vi "RedMoRaceTiming.vi"() -> ()   [LabVIEW 2022 SP3]
uses:
  <vilib>/event_ctls.llb/eventvkey.ctl
  subVIs/BackupFileMgmtStates.ctl
  subVIs/ConfigFileLoopStates.ctl
  <vilib>/Utility/miscctls.llb/LVRowAndColumnUnsignedTypeDef.ctl
  <vilib>/Utility/config.llb/Read Key (I32).vi
  <vilib>/Utility/config.llb/Read Key (Double).vi
  <vilib>/Utility/config.llb/Read Key (Path).vi
  <vilib>/Utility/config.llb/Write Key (Double).vi
  <vilib>/Utility/config.llb/Write Key (I32).vi
  <vilib>/Utility/config.llb/Write Key (Path).vi
  <vilib>/Utility/file.llb/Write Delimited Spreadsheet (string).vi
  <vilib>/Utility/config.llb/NI_LVConfig.lvlib
panel:
  out "Config File Error?":bool
  out "Mode":bool
  out "Event Handler Error?":bool
  out "Backup File Error?":bool
  out "File Mgmt Error?":bool
  out "Finish Table":string[][](table)
  out "Duplicate Bib #s":string[](array[string])
  out "Backup File Saving?":bool
  out "Overall Error Status":bool
  in  "Clear Next Bib":bool
  in  "Bib":string
  out "Race Time":string
  in  "Tab Control":T1(tab)
  out "Racers Remaining":i32
  in  "Enable Button Timing Controls":bool
  out "Duplicate Bib #s":i32
  in  "Bib-Only Button":bool
  in  "Time Only Button":bool
  in  "Control Time Button":bool
  out "Total Times":i32
  out "Total Bibs":i32
  out "Total Control Times":i32
  out "File I/O Error":errorcluster
  out "Backup File I/O Error":errorcluster
  out "Total Racers":i32
  in  "stop":bool
  in  "Time Correction in seconds (increments by .1s)":dbl step=0.1
  out "Overall error out":errorcluster
  in  "Total Racers Control":i32
  in  "Setup/Race Mode Toggle":bool=TRUE
  out "Setup Mode":bool
  out "Race Mode":bool=TRUE
  in  "Save Config File":bool
  in  "CLEAR ARRAYS":bool
  in  "External/Backup Data Path":path=path "D:/RedMoRace"
  in  "SAVE TO FILE":bool
  out "File Path of Main Race File":path
  in  "Enable?":bool=TRUE
  out "Backup File I/O State":T2
  out "ArrayOfControlTimeMarkers":string[](array[string])
  out "VKey":T3
  out "ArrayOfBibs":string[](array[string])
  out "*(type *) &x":string
  out "Char":i16
  out "ArrayOfTimes":string[](array[string])
  # "Red Mo Race Timing\nv2025\nDeveloped by Aaron Fleishman"
  # "Index"
  # "Bib"
  # "Time"
  # "Control Time?"
  # "Statistics"
  # "This is race timing software for downriver canoe and kayak racing. This was designed to operate using a number pad (built-in or USB attachable).\n\nThe software app is able to log three different kinds of data:\n - Time Only - SPACE BAR.\n - Control Time (Bib + Time) - R key\n - Bib only (starting from last control time or last bib, use carefully) - ENTER (on number pad only)"
  # "Timing Controls"
  # "Race Time Correction"
  # "Number of Total Racers Setup"
  # "Errors"
  # "Primary File Management"
  # "External/Backup File Management"
  # "This application is used to assist in timing for the Red Moshannon Downriver Race.\n\n1. Open timing software several minutes prior to finishers and use \"Time/Racer Setup & Errors\" to sync \"Race Time\" in app with official race time stopwatch. Once finishers have crossed the line, do not make any adjustments to time.\n\n2. Configure backup file. The app will store two copies of the race data, one locally and one in a backup location. Typically, the backup location is a remote drive or SD card. This provides backup in case the PC has sudden failure.\n\n3. If known, update the total number of boats racing. This will give you a countdown of total bibs remaining on the main screen.\n\n4. For operations, you need to have multiple spotters. The spotters should have notepads ready to record bib numbers in order that they cross the finish line.\n\n5. As timer, your primary responsbility is to log TIMES. The spotters primary responsbility is to log BIBS in the correct order. After the race, you can merge the two.\n\n6. In order to reduce a single missed value messing all of the data, the timers and spotters should employ \"Control Times\" as frequently as able. Control Times are known correct bib + correct time. If a single boat is crossing with plenty of time before and after, queue the bib number in the box using the number keys, and use the \"R\" key when the boater crosses the line to log a control time. Spotters should also record the time with bib number.\n\n7. After the race, you need to go back and fill in the gaps between Control Times with missing bib numbers. \n\n8. During the race, if you log a couple times without bib #s, you may enter missing bibs in chronological order but only from  the last empty spot or control time. You must use a keypad Enter button to use this feature. Be careful using it. Merging bib numbers with your spotter post-race is preferred.\n\n9. After race, combine timing application output with registration and start times to generate full race results."
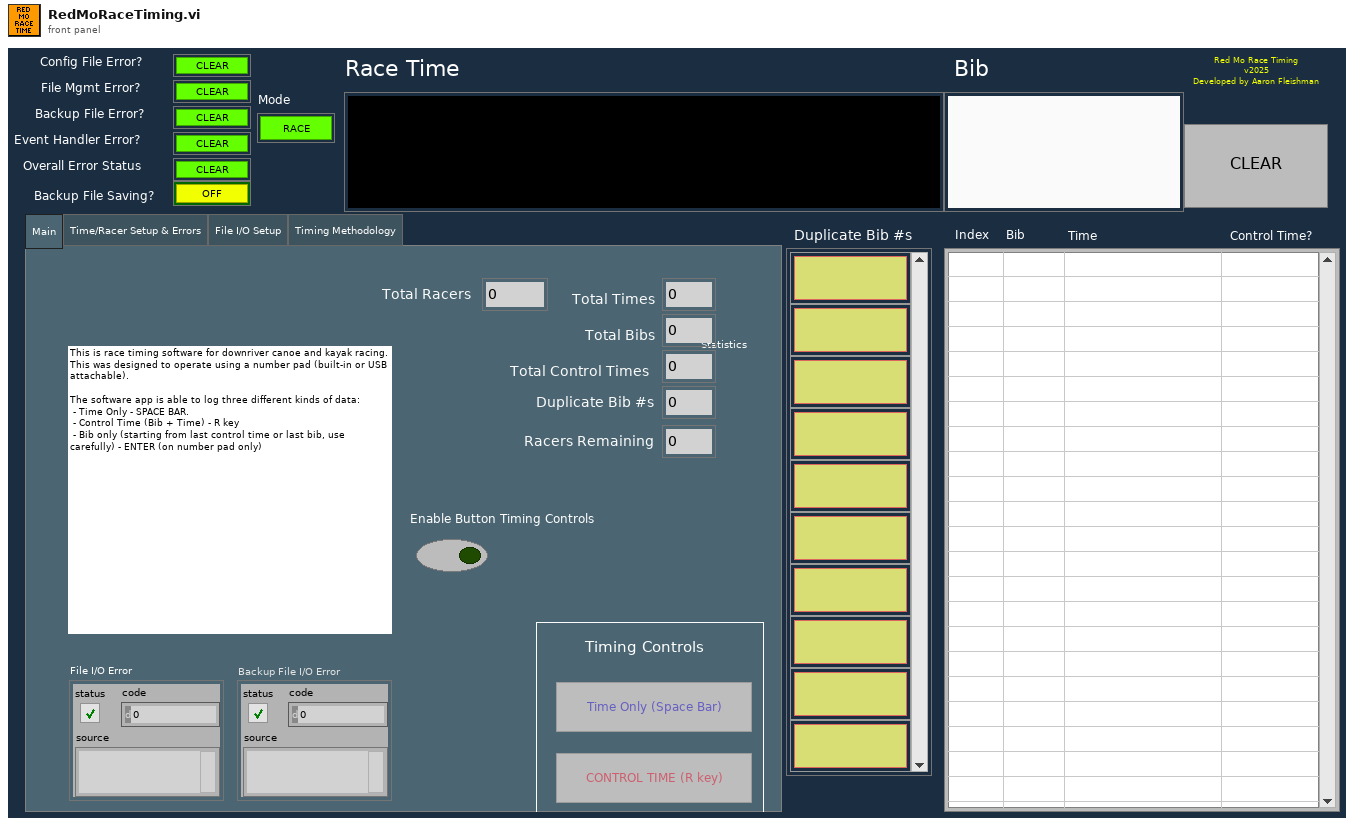
[diagram p1: front panel]
types:
  T1 = enum32{"Main", "Time/Racer Setup & Errors", "File I/O Setup", "Timing Methodology"}
  T2 = typedef "BackupFileMgmtStates.ctl" = enum16{"Idle", "Open File Reference", "Save", "Exit"}
  T3 = typedef "eventvkey.ctl" = enum16{"ASCII", "Enter", "Return", "Shift", "Ctrl", "Alt", "Cmd", "Opt", "Caps", "NumLock", "Clear", "Break", "Up", "Down", "Left", "Right", "Insert", "Delete", "Home", "End", "PageUp", "PageDown", "Escape", "Help", "Pause", "ScrollLock", "F1", "F2", "F3", "F4", "F5", "F6", "F7", "F8", "F9", "F10", "F11", "F12", "F13", "F14", "F15", "F16", "F17", "F18", "F19", "F20", "F21", "F22", "F23", "F24", "Play", "VolumeUp", "VolumeDown", "Mute", "Two Byte Char"}
  T4 = typedef "ConfigFileLoopStates.ctl" = enum16{"Idle", "Read Config File", "Save Config File"}
  T5 = typedef "LVRowAndColumnUnsignedTypeDef.ctl" = cluster{"Row":u32, "Column":u32}
  T6 = enum8{"Enabled", "Disabled", "Disabled and Grayed Out"}
  T7 = typedef "NI_LVConfig.lvlib/Config Data RefNum.ctl" = refnum<k1>
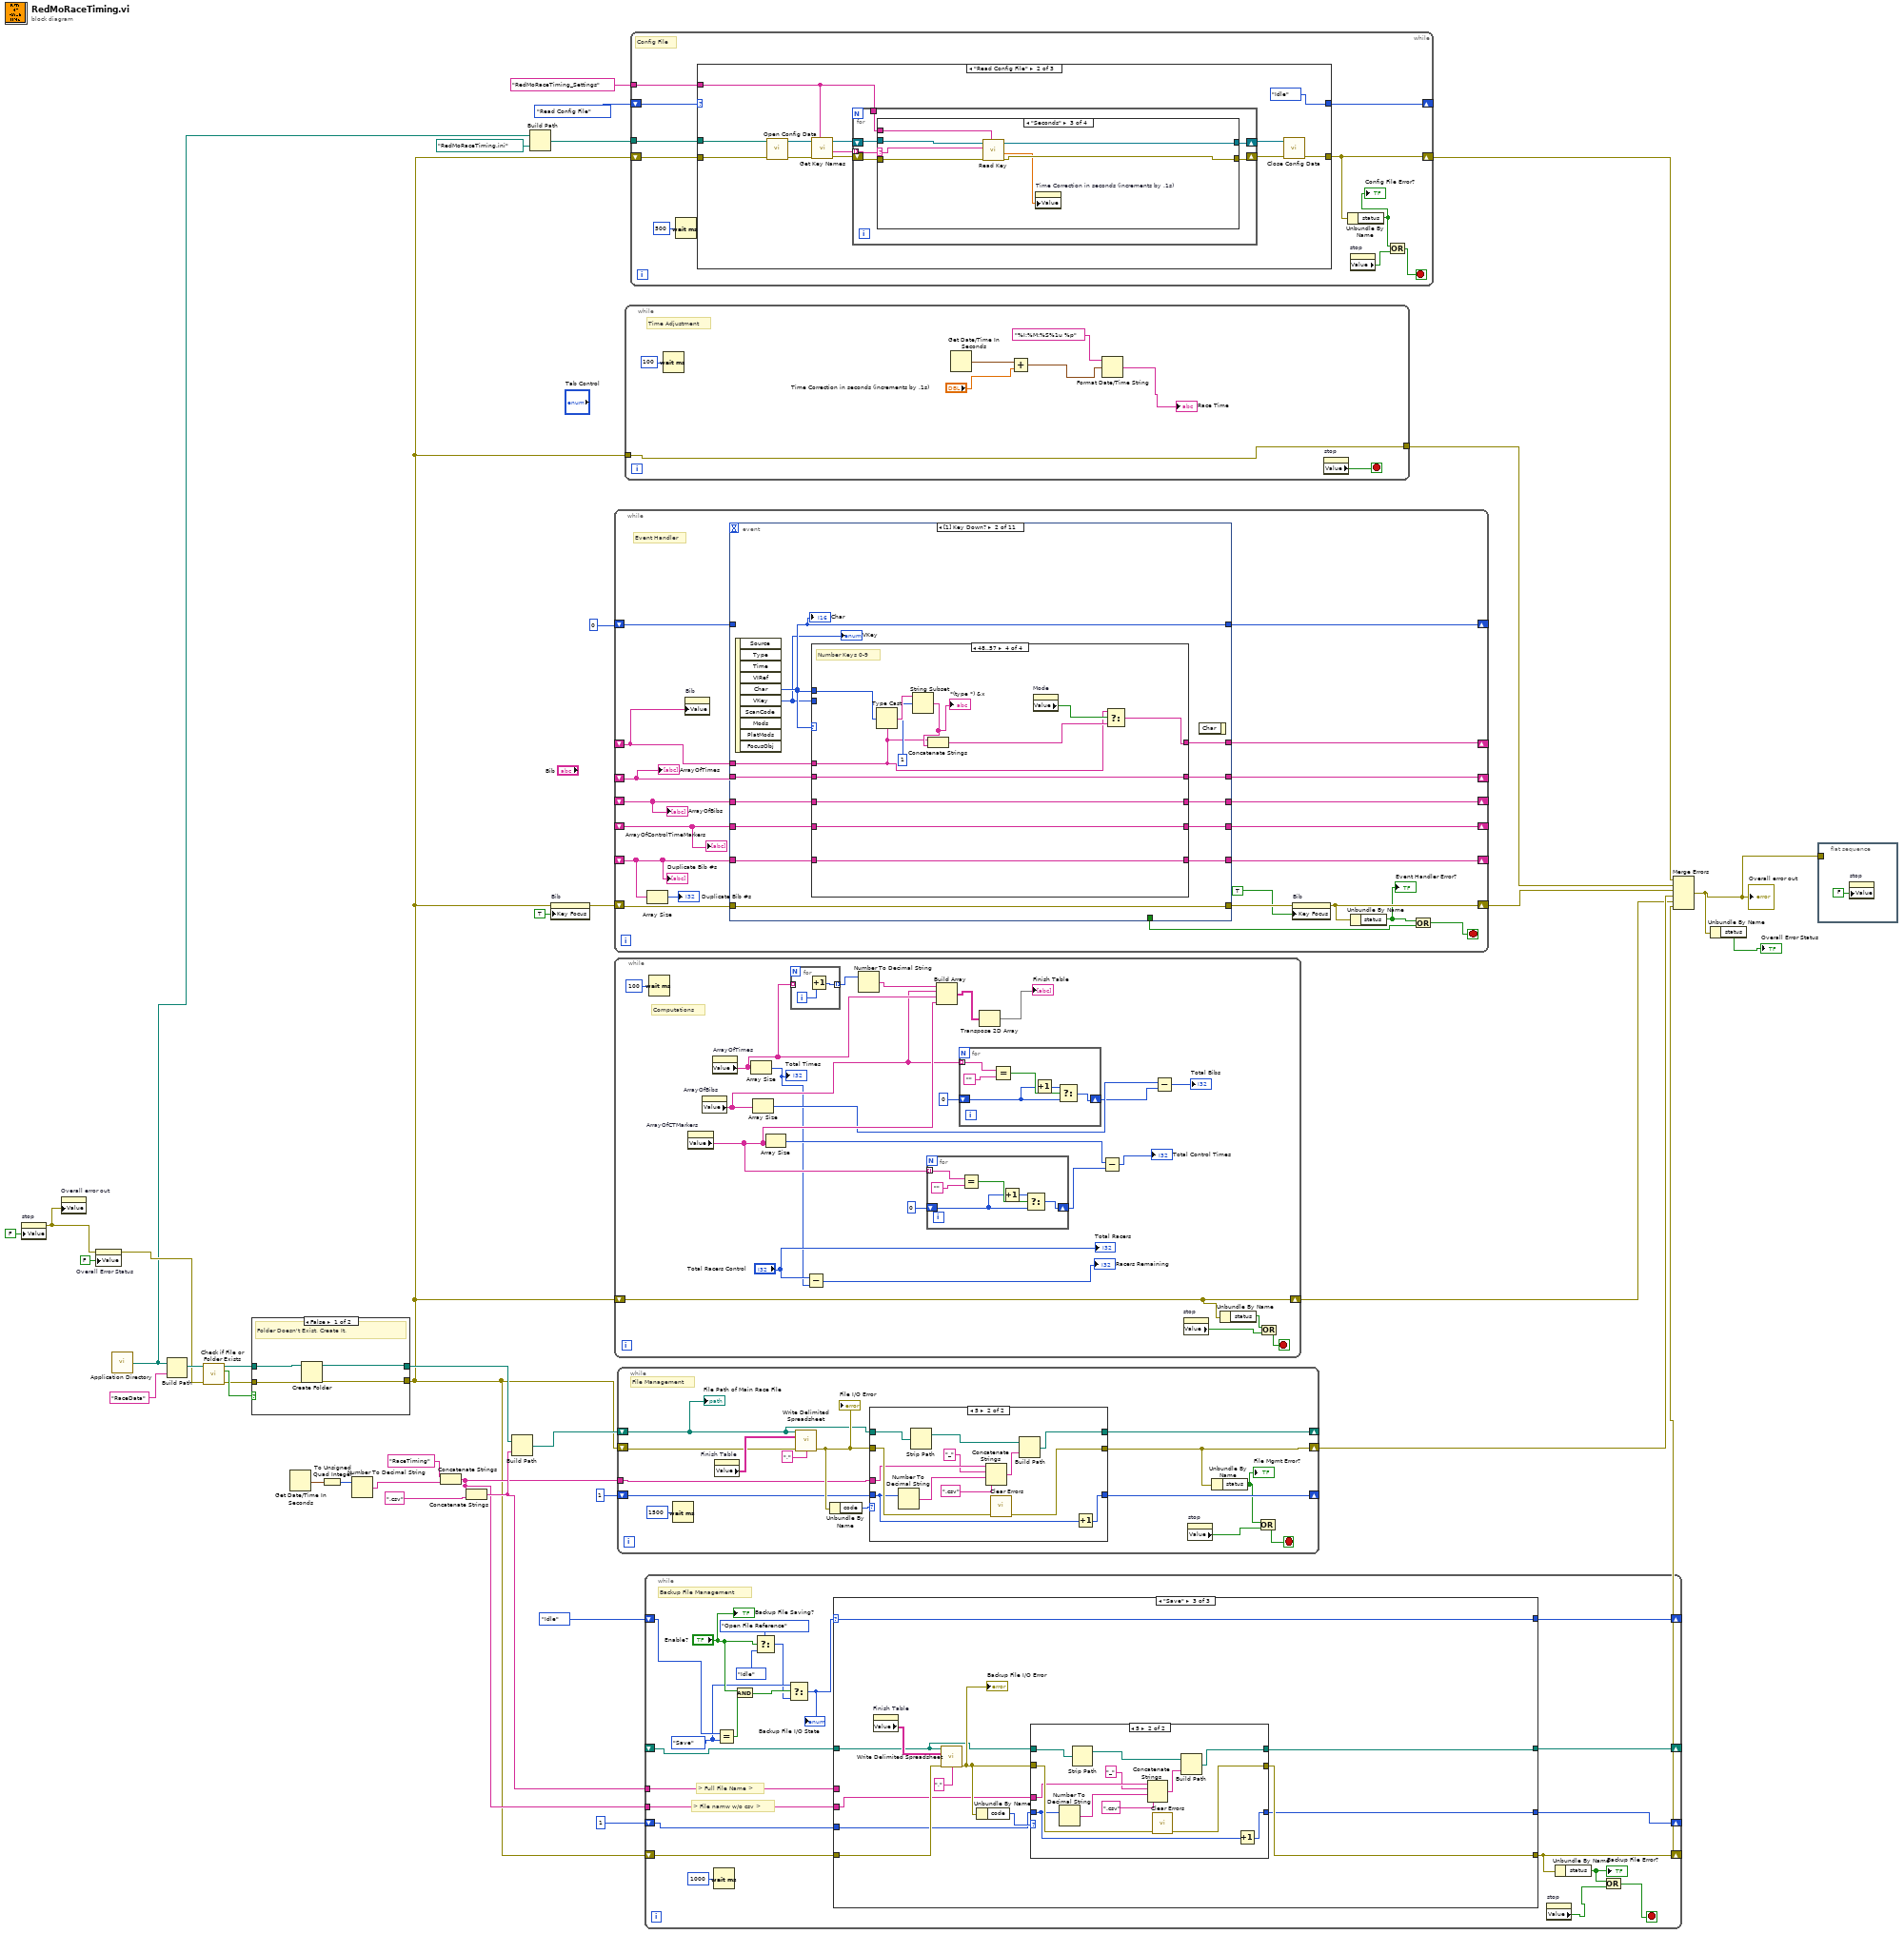
[diagram p0: block diagram]
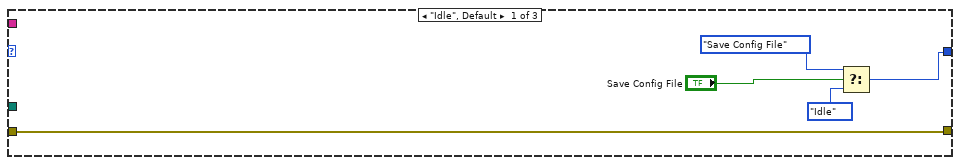
[diagram p2: hidden frame]
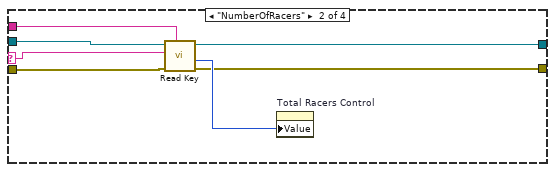
[diagram p4: hidden frame]
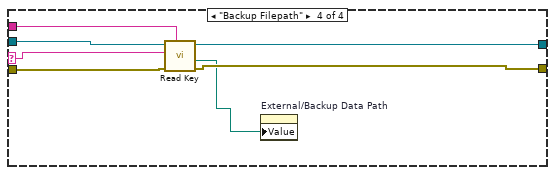
[diagram p5: hidden frame]
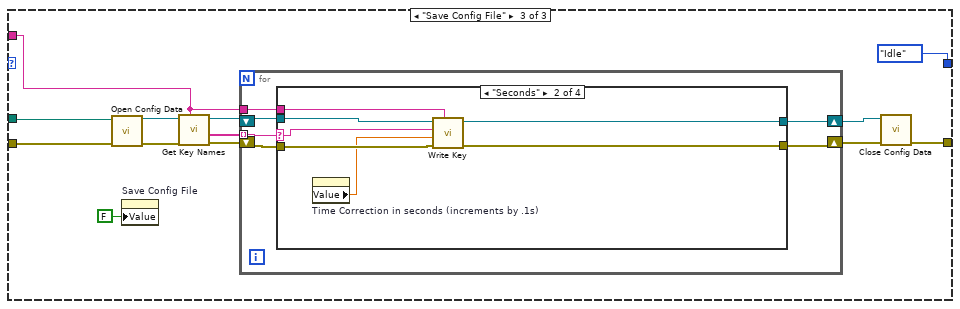
[diagram p6: hidden frame]
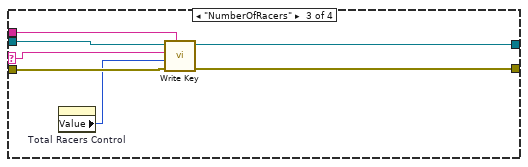
[diagram p8: hidden frame]
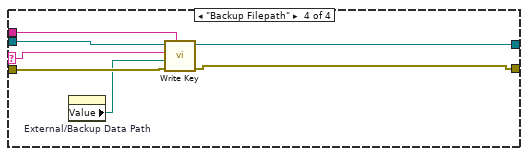
[diagram p9: hidden frame]
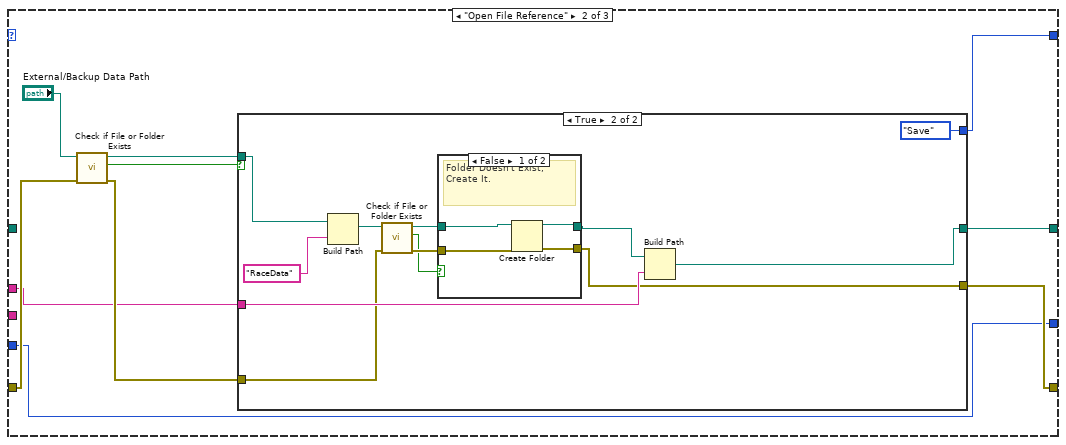
[diagram p11: hidden frame]
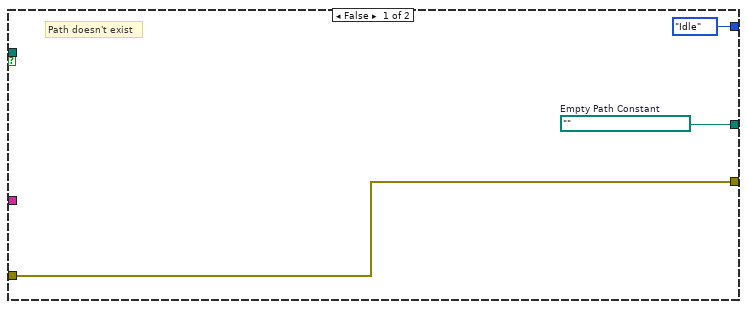
[diagram p12: hidden frame]
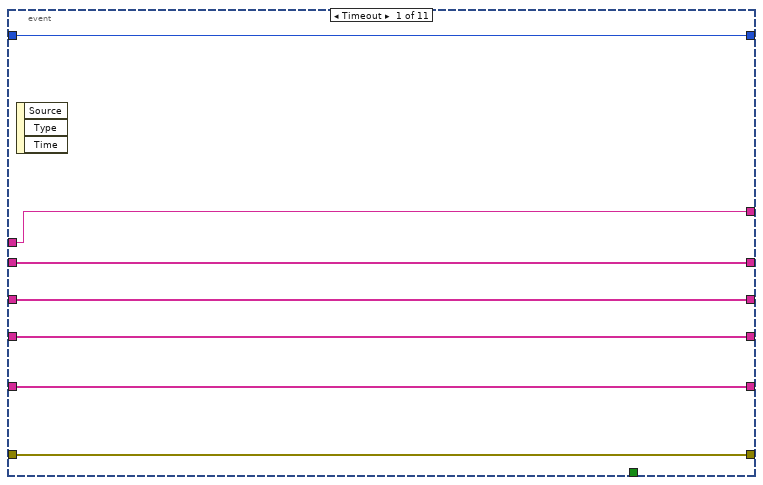
[diagram p17: hidden frame]
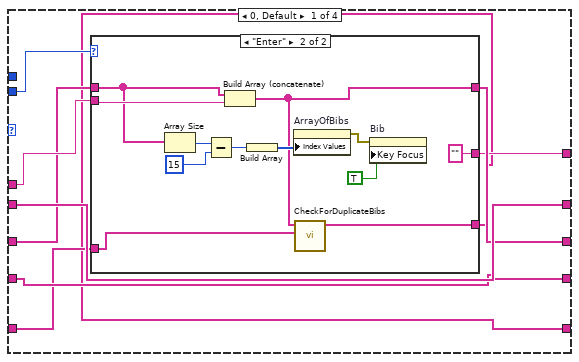
[diagram p18: hidden frame]
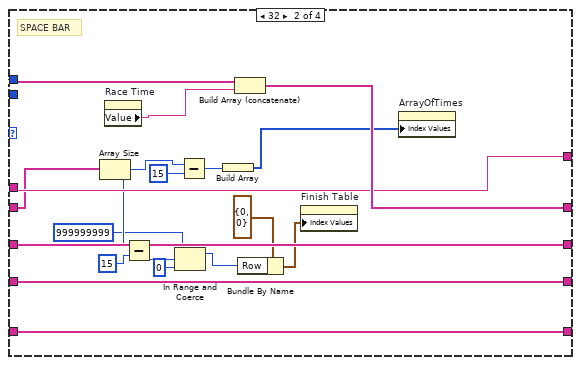
[diagram p20: hidden frame]
diagram:
  n1 = property on="stop" class="Bool (strict)"("Value"=FALSE ("stop")) -> (error out=w15:errorcluster)  [unwired: 2 in, 1 out]
  n2 = property on="Overall error out" class="Clust (strict)"("Value"=w15) -> ()  [unwired: 2 in, 2 out]
  n3 = property on="Overall Error Status" class="Bool (strict)"(error in=w15, "Value"=FALSE ("Error Status")) -> (error out=w8:errorcluster)  [unwired: 1 in, 1 out]
  n4 = call <vilib>:"Application Directory.vi"() -> ("Application Directory"=w7:path)
  n5 = Build Path(base path=w7, name or relative path="RaceData") -> (appended path=w31:path)
  n6 = call <vilib>:"Check if File or Folder Exists.vi"("error in (no error)"=w8, "path"=w31) -> ("error out"=w27:errorcluster, "file or folder exists?"=w30:bool, "dup path"=w29:path)  [unwired: 7 in]
  n7 = case shown="False" w30 {
    tunnel: w29 -> [w42 w44]
    tunnel: [w39 w44] -> w28
    tunnel: w27 -> [w41 w43]
    tunnel: [w40 w43] -> w3
    frame False {
      # "Folder Doesn't Exist, Create It."
      n8 = Create Folder(path (use dialog)=w42, error in=w41) -> (created path=w39:path, error out=w40:errorcluster)  [unwired: 1 in, 1 out]
    }
    frame True {
      # "Folder Exists"
    }
  }
  n9 = Get Date/Time In Seconds() -> (seconds since 1Jan1904=w36:timestamp)
  n10 = To Unsigned Quad Integer(1:w36) -> (0:w35:u64)
  n11 = Number To Decimal String(number=w35) -> (decimal integer string=w34:string)  [unwired: 1 in]
  n12 = Concatenate Strings("RaceTiming", w34) -> (w10:string)
  n13 = Concatenate Strings(w10, ".csv") -> (w12:string)
  n14 = Build Path(base path=w28, name or relative path=w12) -> (appended path=w33:path)
  n15 = Build Path(base path=w7, name or relative path=path "RedMoRaceTiming.ini") -> (appended path=w5:path)
  n16 = property on="Bib" class="Str"(error in=w3, "Key Focus"=TRUE) -> (error out=w25:errorcluster)  [unwired: 1 in, 1 out]
  n17 = while {
    shift-right: [w63] -> _
    shift-left: i16 0 ("Char") -> [w64]
    shift-right: [w62] -> _
    shift-left: _ -> [w61]
    shift-right: [w60] -> _
    shift-left: _ -> [w59]
    shift-right: [w57] -> _
    shift-left: _ -> [w58]
    shift-right: [w54] -> _
    shift-left: _ -> [w55]
    shift-right: [w53] -> _
    shift-left: _ -> [w46]
    shift-right: [w50] -> w23
    shift-left: w25 -> [w49]
    stop <- w51 stop-if-true
    # "Event Handler"
    n18 = Array Size(array=w46) -> (size(s)=→"Duplicate Bib #s":i32)
    n19 = property on="Bib" class="Str"("Value"=w59) -> ()  [unwired: 2 in, 2 out]
    n20 = event shown="[1] Key Down?" {
      selector: _ -> [_ _ _ _ _ _ _ _ _ _ _]
      dyn-events: _ -> [_ _ _ _ _ _ _ _ _ _ _]
      timeout: _ -> [_ _ _ _ _ _ _ _ _ _ _]
      tunnel: w64 -> [w71 _ w180 w207 w223 w245 w269 w294 w311 w321 w332]
      tunnel: [w71 w77 w180 w207 w223 w245 w269 w294 w311 w321 w332] -> w63
      tunnel: w49 -> [w70 w84 w177 w216 w217 w255 w281 w288 w305 w317 w329]
      tunnel: [w70 w84 w176 w216 w217 w255 w281 w288 w305 w316 w328] -> w56
      tunnel: w61 -> [w69 w83 w198 w215 w221 w254 w271 w292 w309 w323 w333]
      tunnel: [w69 w82 w197 w215 w221 w253 w270 w292 w309 w323 w333] -> w62
      tunnel: w59 -> [w66 w81 w196 w214 w222 _ w282 w293 w310 w322 _]
      tunnel: [w66 w80 w196 "" ("Bib Number") w222 "" ("Bib Number") w282 w293 w310 w322 "" ("Bib Number")] -> w60
      tunnel: w58 -> [w67 w79 w195 w212 w220 w251 w273 w291 w308 w324 w334]
      tunnel: [w67 w78 w195 w211 w220 w250 w272 w291 w308 w324 w334] -> w57
      tunnel: w55 -> [w68 w75 w194 w210 w219 w249 w275 w290 w307 w325 w335]
      tunnel: [w68 w74 w194 w210 w219 w248 w266 w290 w307 w325 w335] -> w54
      tunnel: w46 -> [w65 w73 w193 w209 w218 w247 w268 w289 w306 w312 w330]
      tunnel: [w65 w72 w193 w208 w218 w246 w267 w289 w306 w312 w330] -> w53
      tunnel: [_ _ _ _ "stop" _ _ _ _ _ _] -> w48
      event Timeout {
        n21 = event-data() -> ()  [unwired: 1 in, 3 out]
      }
      event Key Down? {
        n22 = event-data() -> ("Char"=w77:i16, "VKey"=w76:T3)  [unwired: 1 in, 8 out]
        "Char" <- w77
        "VKey" <- w76
        n23 = case shown="48..57" w77 {
          tunnel: w83 -> [w93 w121 w149 w175]
          tunnel: [w93 w126 w153 w175] -> w82
          tunnel: w81 -> [w91 w125 _ w165]
          tunnel: w77 -> [_ _ _ w174]
          tunnel: [w88 w125 "" ("Bib Number") w164] -> w80
          tunnel: w79 -> [w90 w124 w147 w170]
          tunnel: [w89 w124 w138 w170] -> w78
          tunnel: w76 -> [w92 _ _ _]
          tunnel: w75 -> [w87 w120 w143 w169]
          tunnel: [w87 w120 w141 w169] -> w74
          tunnel: w73 -> [w86 w110 w140 w168]
          tunnel: [w85 w110 w139 w168] -> w72
          frame 0, Default {
            n24 = case shown="\"Enter\"" w92 {
              tunnel: w90 -> [w96 w106]
              tunnel: w91 -> [w95 w108]
              tunnel: [w96 w98] -> w89
              tunnel: [w95 "" ("Bib Number")] -> w88
              tunnel: w86 -> [w94 w99]
              tunnel: [w94 w97] -> w85
              frame Default {
              }
              frame "Enter" {
                n25 = Array Size(array=w106) -> (size(s)=w105:i32)
                n26 = Subtract(x=w105, y=15) -> (x-y=w102:i32)
                n27 = Build Array (concatenate)(w106, w108) -> (w98:string[])
                n28 = Build Array(w102) -> (w103:i32[])
                n29 = property on="ArrayOfBibs" class="Arr (strict)"("Index Values"=w103) -> (error out=w100:errorcluster)  [unwired: 2 in, 1 out]
                n30 = call "CheckForDuplicateBibs.vi"("ArrayOfDuplicateBibNumbers"=w99, "ArrayOfBibs"=w98) -> ("ArrayOfDuplicateBibNumbers"=w97:string[])  [unwired: 9 in]
                n31 = property on="Bib" class="Str"(error in=w100, "Key Focus"=TRUE) -> ()  [unwired: 1 in, 2 out]
              }
            }
          }
          frame 32 {
            # "SPACE BAR"
            n32 = Array Size(array=w121) -> (size(s)=w116:i32)
            n33 = property on="Race Time" class="Str"() -> ("Value"=w109:string)  [unwired: 2 in, 2 out]
            n34 = Subtract(x=w116, y=15) -> (x-y=w114:i32)
            n35 = In Range and Coerce(upper limit=999999999, x=w114, lower limit=0) -> (coerced(x)=w112:i32)  [unwired: 1 out]
            n36 = Subtract(x=w116, y=15) -> (x-y=w122:i32)
            n37 = Build Array(w122) -> (w123:i32[])
            n38 = Build Array (concatenate)(w121, w109) -> (w126:string[])
            n39 = Bundle By Name(cluster=T5 {"Row"=0, "Column"=0} ("Index Values"), "Row"=w112) -> (w117:T5)
            n40 = property on="Finish Table" class="Tbl (strict)"("Index Values"=w117) -> ()  [unwired: 2 in, 2 out]
            n41 = property on="ArrayOfTimes" class="Arr (strict)"("Index Values"=w123) -> ()  [unwired: 2 in, 2 out]
          }
          frame 114 {
            # "\"R\" (Control Time)"
            n42 = property on="Bib" class="Str"() -> ("Value"=w128:string)  [unwired: 2 in, 2 out]
            n43 = Array Size(array=w149) -> (size(s)=w130:i32)
            n44 = Empty String/Path?(string/path=w128) -> (empty?=w127:bool)
            n45 = Subtract(x=w130, y=15) -> (x-y=w151:i32)
            n46 = Subtract(x=w130, y=15) -> (x-y=w134:i32)
            n47 = Array Size(array=w149) -> (size(s)=w142:i32)
            n48 = case shown="True" w127 {
              tunnel: w143 -> [w158 w163]
              tunnel: w142 -> [_ w160]
              tunnel: [w158 w159] -> w141
              frame True {
              }
              frame False {
                n49 = Reshape Array(w163, w160) -> (w161:string[])
                n50 = Insert Into Array(array=w161, index=w160, new element="*") -> (w159:string[])
              }
            }
            n51 = Reshape Array(w147, w142) -> (w146:string[])
            n52 = property on="Race Time" class="Str"() -> ("Value"=w129:string)  [unwired: 2 in, 2 out]
            n53 = In Range and Coerce(upper limit=999999999, x=w134, lower limit=0) -> (coerced(x)=w132:i32)  [unwired: 1 out]
            n54 = Build Array(w151) -> (w152:i32[])
            n55 = Build Array (concatenate)(w149, w129) -> (w153:string[])
            n56 = property on="ArrayOfTimes" class="Arr (strict)"("Index Values"=w152) -> (error out=w144:errorcluster)  [unwired: 2 in, 1 out]
            n57 = Bundle By Name(cluster=T5 {"Row"=0, "Column"=0} ("Index Values"), "Row"=w132) -> (w135:T5)
            n58 = Insert Into Array(array=w146, index=w142, new element=w128) -> (w138:string[])
            n59 = property on="Finish Table" class="Tbl (strict)"("Index Values"=w135) -> ()  [unwired: 2 in, 2 out]
            n60 = property on="Bib" class="Str"(error in=w144, "Key Focus"=TRUE) -> ()  [unwired: 1 in, 2 out]
            n61 = case shown="True" w127 {
              tunnel: w140 -> [w156 w157]
              tunnel: [w155 w157] -> w139
              tunnel: w138 -> [w154 _]
              frame False {
                n62 = call "CheckForDuplicateBibs.vi"("ArrayOfDuplicateBibNumbers"=w156, "ArrayOfBibs"=w154) -> ("ArrayOfDuplicateBibNumbers"=w155:string[])  [unwired: 9 in]
              }
              frame True {
              }
            }
          }
          frame 48..57 {
            # "Number Keys 0-9"
            n63 = Type Cast(type=w165, x=w174) -> (*(type *) &x=w173:string)
            n64 = String Subset(string=w173, offset (0)=1) -> (substring=w171:string)  [unwired: 1 in]
            "*(type *) &x" <- w171
            n65 = Concatenate Strings(w165, w171) -> (w166:string)
            n66 = property on="Mode" class="Bool (strict)"() -> ("Value"=w167:bool)  [unwired: 2 in, 2 out]
            n67 = Select(t=w165, s=w167, f=w166) -> (s? t:f=w164:string)
          }
        }
        n68 = event-data() -> ()  [unwired: 2 in, 1 out]
      }
      event "Time Only Button": Value Change {
        # "SPACE BAR"
        n69 = event-data() -> ("CtlRef"=w179:refnum<vi>)  [unwired: 1 in, 5 out]
        n70 = property class="Bool (strict)"(reference=w179, error in=w177, "Value"=FALSE) -> (error out=w176:errorcluster)  [unwired: 1 out]
        n71 = Array Size(array=w198) -> (size(s)=w187:i32)
        n72 = property on="Race Time" class="Str"() -> ("Value"=w181:string)  [unwired: 2 in, 2 out]
        n73 = Subtract(x=w187, y=15) -> (x-y=w185:i32)
        n74 = In Range and Coerce(upper limit=999999999, x=w185, lower limit=0) -> (coerced(x)=w183:i32)  [unwired: 1 out]
        n75 = Subtract(x=w187, y=15) -> (x-y=w191:i32)
        n76 = Build Array(w191) -> (w192:i32[])
        n77 = Build Array (concatenate)(w198, w181) -> (w197:string[])
        n78 = Bundle By Name(cluster=T5 {"Row"=0, "Column"=0} ("Index Values"), "Row"=w183) -> (w188:T5)
        n79 = property on="ArrayOfTimes" class="Arr (strict)"("Index Values"=w192) -> ()  [unwired: 2 in, 2 out]
        n80 = property on="Finish Table" class="Tbl (strict)"("Index Values"=w188) -> ()  [unwired: 2 in, 2 out]
      }
      event "Bib-Only Button": Value Change {
        n81 = event-data() -> ("CtlRef"=w200:refnum<vi>)  [unwired: 1 in, 5 out]
        n82 = property class="Bool (strict)"(reference=w200, "Value"=FALSE) -> ()  [unwired: 1 in, 2 out]
        n83 = Array Size(array=w212) -> (size(s)=w206:i32)
        n84 = Subtract(x=w206, y=15) -> (x-y=w203:i32)
        n85 = Build Array (concatenate)(w212, w214) -> (w211:string[])
        n86 = Build Array(w203) -> (w204:i32[])
        n87 = property on="ArrayOfBibs" class="Arr (strict)"("Index Values"=w204) -> (error out=w201:errorcluster)  [unwired: 2 in, 1 out]
        n88 = call "CheckForDuplicateBibs.vi"("ArrayOfDuplicateBibNumbers"=w209, "ArrayOfBibs"=w211) -> ("ArrayOfDuplicateBibNumbers"=w208:string[])  [unwired: 9 in]
        n89 = property on="Bib" class="Str"(error in=w201, "Key Focus"=TRUE) -> ()  [unwired: 1 in, 2 out]
      }
      event "stop": Value Change {
        n90 = event-data() -> ()  [unwired: 1 in, 6 out]
      }
      event "Control Time Button": Value Change {
        # "\"R\" (Control Time)"
        n91 = event-data() -> ("CtlRef"=w228:refnum<vi>)  [unwired: 1 in, 5 out]
        n92 = property on="Bib" class="Str"() -> ("Value"=w226:string)  [unwired: 2 in, 2 out]
        n93 = property class="Bool (strict)"(reference=w228, "Value"=FALSE) -> ()  [unwired: 1 in, 2 out]
        n94 = Array Size(array=w254) -> (size(s)=w238:i32)
        n95 = Empty String/Path?(string/path=w226) -> (empty?=w225:bool)
        n96 = Array Size(array=w254) -> (size(s)=w230:i32)
        n97 = property on="Race Time" class="Str"() -> ("Value"=w229:string)  [unwired: 2 in, 2 out]
        n98 = Subtract(x=w230, y=15) -> (x-y=w243:i32)
        n99 = Reshape Array(w251, w238) -> (w241:string[])
        n100 = Subtract(x=w230, y=15) -> (x-y=w234:i32)
        n101 = case shown="False" w225 {
          tunnel: w249 -> [w264 w265]
          tunnel: [w263 w265] -> w248
          tunnel: w238 -> [w260 _]
          frame False {
            n102 = Reshape Array(w264, w260) -> (w261:string[])
            n103 = Insert Into Array(array=w261, index=w260, new element="*") -> (w263:string[])
          }
          frame True {
          }
        }
        n104 = In Range and Coerce(upper limit=999999999, x=w234, lower limit=0) -> (coerced(x)=w232:i32)  [unwired: 1 out]
        n105 = Build Array(w243) -> (w244:i32[])
        n106 = Build Array (concatenate)(w254, w229) -> (w253:string[])
        n107 = property on="ArrayOfTimes" class="Arr (strict)"("Index Values"=w244) -> (error out=w239:errorcluster)  [unwired: 2 in, 1 out]
        n108 = Bundle By Name(cluster=T5 {"Row"=0, "Column"=0} ("Index Values"), "Row"=w232) -> (w235:T5)
        n109 = Insert Into Array(array=w241, index=w238, new element=w226) -> (w250:string[])
        n110 = property on="Finish Table" class="Tbl (strict)"("Index Values"=w235) -> ()  [unwired: 2 in, 2 out]
        n111 = property on="Bib" class="Str"(error in=w239, "Key Focus"=TRUE) -> ()  [unwired: 1 in, 2 out]
        n112 = case shown="True" w225 {
          tunnel: w250 -> [_ w259]
          tunnel: w247 -> [w256 w258]
          tunnel: [w256 w257] -> w246
          frame True {
          }
          frame False {
            n113 = call "CheckForDuplicateBibs.vi"("ArrayOfDuplicateBibNumbers"=w258, "ArrayOfBibs"=w259) -> ("ArrayOfDuplicateBibNumbers"=w257:string[])  [unwired: 9 in]
          }
        }
      }
      event "CLEAR ARRAYS": Value Change {
        n114 = event-data() -> ("CtlRef"=w280:refnum<vi>)  [unwired: 1 in, 5 out]
        n115 = property class="Bool (strict)"(reference=w280, "Value"=FALSE) -> ()  [unwired: 1 in, 2 out]
        n116 = Two Button Dialog(message="Are you sure you want to CLEAR all the times?", 1:"KEEP" ("F button name (\"Cancel\")"), 2:"CLEAR" ("T button name (\"OK\")")) -> (T button?=w274:bool)
        n117 = case shown="True" w274 {
          tunnel: w275 -> [w283 _]
          tunnel: [w286 w287] -> w272
          tunnel: w273 -> [w286 _]
          tunnel: w271 -> [w285 _]
          tunnel: [w285 w287] -> w270
          tunnel: w268 -> [w284 _]
          tunnel: [w284 w287] -> w267
          tunnel: [w283 w287] -> w266
          frame False {
          }
          frame True {
            w287 = string[] [] ("ArrayOfTimes")
          }
        }
      }
      event "Enable Button Timing Controls": Value Change {
        n118 = event-data() -> ("NewVal"=w295:bool)  [unwired: 1 in, 5 out]
        n119 = Select(t=T6."Enabled" ("Disabled"), s=w295, f=T6."Disabled and Grayed Out" ("Disabled")) -> (s? t:f=w296:T6)
        n120 = property on="Time Only Button" class="Bool (strict)"("DisabledEnum"=w296) -> ()  [unwired: 2 in, 2 out]
        n121 = property on="Control Time Button" class="Bool (strict)"("DisabledEnum"=w296) -> ()  [unwired: 2 in, 2 out]
        n122 = property on="Bib-Only Button" class="Bool (strict)"("DisabledEnum"=w296) -> ()  [unwired: 2 in, 2 out]
      }
      event "Setup/Race Mode Toggle": Value Change {
        w301 = T6."Enabled" ("Disabled")
        w300 = T6."Disabled and Grayed Out" ("Disabled")
        n123 = event-data() -> ("OldVal"=→"Setup Mode" →"Mode":bool, "NewVal"=w302:bool)  [unwired: 1 in, 4 out]
        "Race Mode" <- w302
        n124 = Select(t=w300, s=w302, f=w301) -> (s? t:f=w303:T6)
        n125 = Select(t=w301, s=w302, f=w300) -> (s? t:f=w299:T6)
        n126 = property on="Time Correction in seconds (increments by .1s)" class="DigNum (strict)"("DisabledEnum"=w303) -> ()  [unwired: 2 in, 2 out]
        n127 = property on="Total Racers Control" class="DigNum (strict)"("DisabledEnum"=w303) -> ()  [unwired: 2 in, 2 out]
        n128 = property on="Bib" class="Str"("DisabledEnum"=w299) -> ()  [unwired: 2 in, 2 out]
      }
      event "SAVE TO FILE": Value Change {
        n129 = event-data() -> ("CtlRef"=w327:refnum<vi>)  [unwired: 1 in, 5 out]
        n130 = property class="Bool (strict)"(reference=w327, error in=w317, "Value"=FALSE) -> (error out=w315:errorcluster)  [unwired: 1 out]
        n131 = property on="File Path of Main Race File" class="Path"(error in=w315) -> (error out=w314:errorcluster, "Value"=w320:path)  [unwired: 1 in, 1 out]
        n132 = property on="Finish Table" class="Tbl (strict)"(error in=w314) -> (error out=w313:errorcluster, "Value"=w319:string[][])  [unwired: 1 in, 1 out]
        n133 = call-poly <vilib>:"Write Delimited Spreadsheet.vi"("file path (dialog if empty)"=w320, "2D data"=w319, "error in (no error)"=w313, "delimiter (\\t)"="," ("delimiter (\\t)")) -> ("error out"=w316:errorcluster)  [unwired: 10 in, 1 out]
      }
      event "Clear Next Bib": Value Change {
        n134 = event-data() -> ("CtlRef"=w337:refnum<vi>)  [unwired: 1 in, 5 out]
        n135 = property class="Bool (strict)"(reference=w337, error in=w329, "Value"=FALSE) -> (error out=w328:errorcluster)  [unwired: 1 out]
      }
    }
    n136 = property on="Bib" class="Str"(error in=w56, "Key Focus"=TRUE) -> (error out=w50:errorcluster)  [unwired: 1 in, 1 out]
    n137 = Unbundle By Name(w50) -> ("status"=w47:bool)
    "Event Handler Error?" <- w47
    n138 = Or(x=w47, y=w48) -> (x .or. y?=w51:bool)
    "ArrayOfTimes" <- w61
    "ArrayOfBibs" <- w58
    "ArrayOfControlTimeMarkers" <- w55
    "Duplicate Bib #s" <- w46
  }
  n139 = while {
    shift-right: [w341] -> w19
    shift-left: w3 -> [w341]
    stop <- w338 stop-if-true
    # "Computations"
    n140 = Wait (ms)(milliseconds to wait=u32 100) -> ()  [unwired: 1 out]
    n141 = property on="ArrayOfCTMarkers" class="Arr (strict)"() -> ("Value"=w357:string[])  [unwired: 2 in, 2 out]
    n142 = property on="ArrayOfBibs" class="Arr (strict)"() -> ("Value"=w345:string[])  [unwired: 2 in, 2 out]
    n143 = property on="ArrayOfTimes" class="Arr (strict)"() -> ("Value"=w348:string[])  [unwired: 2 in, 2 out]
    n144 = Array Size(array=w348) -> (size(s)=w343:i32)
    "Total Times" <- w343
    n145 = Array Size(array=w345) -> (size(s)=w351:i32)
    n146 = Array Size(array=w357) -> (size(s)=w355:i32)
    n147 = for {
      tunnel: w348 -> [_] mode=indexing
      tunnel: [w361] -> w347 mode=indexing
      i -> [w362]
      n148 = Increment(x=w362) -> (x+1=w361:i32)
    }
    n149 = Subtract(x="Total Racers Control", y=w343) -> (x-y=→"Racers Remaining":i32)
    n150 = Number To Decimal String(number=w347) -> (decimal integer string=w346:string[])  [unwired: 1 in]
    n151 = for {
      tunnel: w357 -> [w373] mode=indexing
      shift-right: [w371] -> w353
      shift-left: 0 -> [w369]
      n152 = Equal?(x=w373, y="") -> (x = y?=w372:bool)
      n153 = Increment(x=w369) -> (x+1=w370:i32)
      n154 = Select(t=w370, s=w372, f=w369) -> (s? t:f=w371:i32)
    }
    n155 = Build Array(w346, w345, w348, w357) -> (w359:string[][])
    n156 = for {
      tunnel: w345 -> [w367] mode=indexing
      shift-right: [w365] -> w350
      shift-left: 0 -> [w363]
      n157 = Equal?(x=w367, y="") -> (x = y?=w366:bool)
      n158 = Increment(x=w363) -> (x+1=w364:i32)
      n159 = Select(t=w364, s=w366, f=w363) -> (s? t:f=w365:i32)
    }
    n160 = Transpose 2D Array(2D array=w359) -> (transposed array=→"Finish Table":string[][])
    n161 = Subtract(x=w355, y=w353) -> (x-y=→"Total Control Times":i32)
    n162 = Subtract(x=w351, y=w350) -> (x-y=→"Total Bibs":i32)
    n163 = property on="stop" class="Bool (strict)"() -> ("Value"=w339:bool)  [unwired: 2 in, 2 out]
    n164 = Unbundle By Name(w341) -> ("status"=w340:bool)
    n165 = Or(x=w340, y=w339) -> (x .or. y?=w338:bool)
    "Total Racers" <- "Total Racers Control"
  }
  n166 = while {
    shift-right: [w377] -> _
    shift-left: w33 -> [w376]
    shift-right: [w381] -> w20
    shift-left: w3 -> [w386]
    tunnel: w10 -> [w380]
    shift-right: [w378] -> _
    shift-left: u32 1 ("milliseconds to wait") -> [w379]
    stop <- w385 stop-if-true
    # "File Management"
    n167 = Wait (ms)(milliseconds to wait=u32 1500) -> ()  [unwired: 1 out]
    n168 = property on="Finish Table" class="Tbl (strict)"() -> ("Value"=w388:string[][])  [unwired: 2 in, 2 out]
    n169 = call-poly <vilib>:"Write Delimited Spreadsheet.vi"("file path (dialog if empty)"=w376, "2D data"=w388, "error in (no error)"=w386, "delimiter (\\t)"="," ("delimiter (\\t)")) -> ("error out"=w382:errorcluster)  [unwired: 10 in, 1 out]
    "File I/O Error" <- w382
    n170 = Unbundle By Name(w382) -> ("code"=w383:i32)
    n171 = case shown="5" w383 {
      tunnel: w382 -> [w391 w404]
      tunnel: [w391 w403] -> w381
      tunnel: w376 -> [w392 w402]
      tunnel: w380 -> [_ w398]
      tunnel: w379 -> [w390 w399]
      tunnel: [w390 w400] -> w378
      tunnel: [w392 w393] -> w377
      frame 0, Default {
      }
      frame 5 {
        n172 = Number To Decimal String(number=w399) -> (decimal integer string=w396:string)  [unwired: 1 in]
        n173 = Strip Path(path=w402) -> (stripped path=w401:path)  [unwired: 1 out]
        n174 = Concatenate Strings(w398, "_" ("string"), w396, ".csv" ("string")) -> (w394:string)
        n175 = call <vilib>:"Clear Errors.vi"("error in (no error)"=w404) -> ("error out"=w403:errorcluster)  [unwired: 5 in, 1 out]
        n176 = Build Path(base path=w401, name or relative path=w394) -> (appended path=w393:path)
        n177 = Increment(x=w399) -> (x+1=w400:u32)
      }
    }
    n178 = property on="stop" class="Bool (strict)"() -> ("Value"=w384:bool)  [unwired: 2 in, 2 out]
    n179 = Unbundle By Name(w381) -> ("status"=w375:bool)
    "File Mgmt Error?" <- w375
    n180 = Or(x=w375, y=w384) -> (x .or. y?=w385:bool)
    "File Path of Main Race File" <- w376
  }
  n181 = while {
    tunnel: w3 -> [w411]
    tunnel: [w411] -> w18
    stop <- w410 stop-if-true
    # "Time Adjustment"
    n182 = Wait (ms)(milliseconds to wait=u32 100) -> ()  [unwired: 1 out]
    n183 = Get Date/Time In Seconds() -> (seconds since 1Jan1904=w407:timestamp)
    n184 = Add(x=w407, y="Time Correction in seconds (increments by .1s)") -> (x+y=w405:timestamp)
    n185 = Format Date/Time String(time format string (%c)="%I:%M:%S%1u %p", seconds (now)=w405) -> (date/time string=→"Race Time":string)  [unwired: 1 in]
    n186 = property on="stop" class="Bool (strict)"() -> ("Value"=w410:bool)  [unwired: 2 in, 2 out]
  }
  n187 = while {
    tunnel: w5 -> [w421]
    shift-right: [w419] -> w2
    shift-left: w3 -> [w420]
    shift-right: [w415] -> _
    shift-left: ConfigFileLoopStates."Read Config File" -> [w422]
    tunnel: "RedMoRaceTiming_Settings" ("section") -> [w413]
    stop <- w417 stop-if-true
    # "Config File"
    n188 = Wait (ms)(milliseconds to wait=u32 500) -> ()  [unwired: 1 out]
    n189 = case shown="\"Read Config File\"" w422 {
      tunnel: w421 -> [_ w439 w481]
      tunnel: w420 -> [w427 w438 w480]
      tunnel: [w427 w430 w471] -> w419
      tunnel: [w423 ConfigFileLoopStates."Idle" ConfigFileLoopStates."Idle"] -> w415
      tunnel: w413 -> [_ w428 w469]
      frame "Idle", Default {
        n190 = Select(t=ConfigFileLoopStates."Save Config File", s="Save Config File", f=ConfigFileLoopStates."Idle") -> (s? t:f=w423:T4)
      }
      frame "Read Config File" {
        n191 = call <vilib>:"Open Config Data.vi"("error in (no error)"=w438, "configuration file path"=w439) -> ("error out"=w436:errorcluster, "refnum"=w437:T7)  [unwired: 7 in, 1 out]
        n192 = call <vilib>:"Get Key Names.vi"("section"=w428, "error in (no error)"=w436, "refnum"=w437) -> ("error out"=w435:errorcluster, "key names"=w434:string[], "refnum out"=w433:T7)  [unwired: 5 in, 1 out]
        n193 = for {
          tunnel: w434 -> [w445] mode=indexing
          shift-right: [w442] -> w429
          shift-left: w433 -> [w444]
          shift-right: [w441] -> w431
          shift-left: w435 -> [w443]
          tunnel: w428 -> [w440]
          n194 = case shown="\"Seconds\"" w445 {
            selector: w445 -> [_ w450 w458 w465]
            tunnel: w444 -> [w447 w454 w461 w468]
            tunnel: w443 -> [w446 w453 w460 w467]
            tunnel: [w447 w451 w459 w466] -> w442
            tunnel: [w446 w449 w457 w464] -> w441
            tunnel: w440 -> [_ w448 w456 w463]
            frame "False", Default {
            }
            frame "NumberOfRacers" {
              n195 = call-poly <vilib>:"Read Key.vi"("section"=w448, "error in (no error)"=w453, "key"=w450, "refnum"=w454) -> ("error out"=w449:errorcluster, "value"=w452:i32, "refnum out"=w451:T7)  [unwired: 4 in, 1 out]
              n196 = property on="Total Racers Control" class="DigNum (strict)"("Value"=w452) -> ()  [unwired: 2 in, 2 out]
            }
            frame "Seconds" {
              n197 = call-poly <vilib>:"Read Key.vi"("section"=w456, "error in (no error)"=w460, "key"=w458, "refnum"=w461) -> ("error out"=w457:errorcluster, "value"=w455:dbl, "refnum out"=w459:T7)  [unwired: 4 in, 1 out]
              n198 = property on="Time Correction in seconds (increments by .1s)" class="DigNum (strict)"("Value"=w455) -> ()  [unwired: 2 in, 2 out]
            }
            frame "Backup Filepath" {
              n199 = call-poly <vilib>:"Read Key.vi"("section"=w463, "error in (no error)"=w467, "key"=w465, "refnum"=w468) -> ("error out"=w464:errorcluster, "value"=w462:path, "refnum out"=w466:T7)  [unwired: 4 in, 1 out]
              n200 = property on="External/Backup Data Path" class="Path"("Value"=w462) -> ()  [unwired: 2 in, 2 out]
            }
          }
        }
        n201 = call <vilib>:"Close Config Data.vi"("error in (no error)"=w431, "refnum"=w429) -> ("error out"=w430:errorcluster)  [unwired: 8 in, 1 out]
      }
      frame "Save Config File" {
        n202 = call <vilib>:"Open Config Data.vi"("error in (no error)"=w480, "configuration file path"=w481) -> ("error out"=w478:errorcluster, "refnum"=w479:T7)  [unwired: 7 in, 1 out]
        n203 = property on="Save Config File" class="Bool (strict)"("Value"=FALSE ("Save Config File")) -> ()  [unwired: 2 in, 2 out]
        n204 = call <vilib>:"Get Key Names.vi"("section"=w469, "error in (no error)"=w478, "refnum"=w479) -> ("error out"=w477:errorcluster, "key names"=w476:string[], "refnum out"=w475:T7)  [unwired: 5 in, 1 out]
        n205 = for {
          tunnel: w476 -> [w487] mode=indexing
          shift-right: [w484] -> w470
          shift-left: w475 -> [w486]
          shift-right: [w483] -> w472
          shift-left: w477 -> [w485]
          tunnel: w469 -> [w482]
          n206 = case shown="\"Seconds\"" w487 {
            selector: w487 -> [_ w493 w500 w507]
            tunnel: w486 -> [w489 w496 w503 w510]
            tunnel: w485 -> [w488 w495 w502 w509]
            tunnel: [w489 w494 w501 w508] -> w484
            tunnel: [w488 w492 w499 w506] -> w483
            tunnel: w482 -> [_ w490 w497 w505]
            frame "False", Default {
            }
            frame "Seconds" {
              n207 = property on="Time Correction in seconds (increments by .1s)" class="DigNum (strict)"() -> ("Value"=w491:dbl)  [unwired: 2 in, 2 out]
              n208 = call-poly <vilib>:"Write Key.vi"("section"=w490, "error in (no error)"=w495, "value"=w491, "key"=w493, "refnum"=w496) -> ("error out"=w492:errorcluster, "refnum out"=w494:T7)  [unwired: 4 in, 1 out]
            }
            frame "NumberOfRacers" {
              n209 = property on="Total Racers Control" class="DigNum (strict)"() -> ("Value"=w498:i32)  [unwired: 2 in, 2 out]
              n210 = call-poly <vilib>:"Write Key.vi"("section"=w497, "error in (no error)"=w502, "value"=w498, "key"=w500, "refnum"=w503) -> ("error out"=w499:errorcluster, "refnum out"=w501:T7)  [unwired: 4 in, 1 out]
            }
            frame "Backup Filepath" {
              n211 = property on="External/Backup Data Path" class="Path"() -> ("Value"=w504:path)  [unwired: 2 in, 2 out]
              n212 = call-poly <vilib>:"Write Key.vi"("section"=w505, "error in (no error)"=w509, "value"=w504, "key"=w507, "refnum"=w510) -> ("error out"=w506:errorcluster, "refnum out"=w508:T7)  [unwired: 4 in, 1 out]
            }
          }
        }
        n213 = call <vilib>:"Close Config Data.vi"("error in (no error)"=w472, "refnum"=w470) -> ("error out"=w471:errorcluster)  [unwired: 8 in, 1 out]
      }
    }
    n214 = Unbundle By Name(w419) -> ("status"=w416:bool)
    "Config File Error?" <- w416
    n215 = property on="stop" class="Bool (strict)"() -> ("Value"=w418:bool)  [unwired: 2 in, 2 out]
    n216 = Or(x=w416, y=w418) -> (x .or. y?=w417:bool)
  }
  n217 = while {
    shift-right: [w523] -> _
    shift-left: BackupFileMgmtStates."Idle" -> [w531]
    shift-right: [w521] -> _
    shift-left: _ -> [w520]
    tunnel: w12 -> [w519]
    shift-right: [w517] -> w22
    shift-left: w3 -> [w518]
    tunnel: w10 -> [w514]
    shift-right: [w512] -> _
    shift-left: u32 1 ("milliseconds to wait") -> [w513]
    stop <- w516 stop-if-true
    w527 = BackupFileMgmtStates."Save" ("y")
    # "> File namw w/o csv >"
    # "> Full File Name >"
    # "Backup File Management"
    n218 = Wait (ms)(milliseconds to wait=u32 1000) -> ()  [unwired: 1 out]
    n219 = Equal?(x=w531, y=w527) -> (x = y?=w530:bool)
    n220 = And(x="Enable?", y=w530) -> (x .and. y?=w528:bool)
    n221 = Select(t=BackupFileMgmtStates."Open File Reference", s="Enable?", f=BackupFileMgmtStates."Idle") -> (s? t:f=w525:T2)
    n222 = Select(t=w527, s=w528, f=w525) -> (s? t:f=w524:T2)
    "Backup File I/O State" <- w524
    n223 = case shown="\"Save\"" w524 {
      selector: w524 -> [w536 _ w579]
      tunnel: [w536 w542 w579] -> w523
      tunnel: w518 -> [w534 w545 w576]
      tunnel: [w535 w540 w571] -> w521
      tunnel: w520 -> [w535 _ w572]
      tunnel: w519 -> [_ w539 _]
      tunnel: [w534 w538 w574] -> w517
      tunnel: w514 -> [_ _ w573]
      tunnel: w513 -> [w533 w537 w569]
      tunnel: [w533 w537 w568] -> w512
      frame "Idle", Default {
      }
      frame "Open File Reference" {
        n224 = call <vilib>:"Check if File or Folder Exists.vi"("error in (no error)"=w545, "path"="External/Backup Data Path") -> ("error out"=w543:errorcluster, "file or folder exists?"=w544:bool, "dup path"=w541:path)  [unwired: 7 in]
        n225 = case shown="True" w544 {
          tunnel: w543 -> [w547 w552]
          tunnel: [BackupFileMgmtStates."Idle" BackupFileMgmtStates."Save"] -> w542
          tunnel: w541 -> [_ w556]
          tunnel: [w548 w553] -> w540
          tunnel: w539 -> [_ w555]
          tunnel: [w547 w551] -> w538
          frame False {
            w548 = path ""  # Empty Path Constant
            # "Path doesn't exist"
          }
          frame True {
            n226 = Build Path(base path=w556, name or relative path="RaceData") -> (appended path=w558:path)
            n227 = call <vilib>:"Check if File or Folder Exists.vi"("error in (no error)"=w552, "path"=w558) -> ("error out"=w561:errorcluster, "file or folder exists?"=w559:bool, "dup path"=w560:path)  [unwired: 7 in]
            n228 = case shown="False" w559 {
              tunnel: w560 -> [w565 w567]
              tunnel: [w562 w567] -> w554
              tunnel: w561 -> [w564 w566]
              tunnel: [w563 w566] -> w551
              frame False {
                # "Folder Doesn't Exist, Create It."
                n229 = Create Folder(path (use dialog)=w565, error in=w564) -> (created path=w562:path, error out=w563:errorcluster)  [unwired: 1 in, 1 out]
              }
              frame True {
                # "Folder Exists"
              }
            }
            n230 = Build Path(base path=w554, name or relative path=w555) -> (appended path=w553:path)
          }
        }
      }
      frame "Save" {
        n231 = property on="Finish Table" class="Tbl (strict)"() -> ("Value"=w577:string[][])  [unwired: 2 in, 2 out]
        n232 = call-poly <vilib>:"Write Delimited Spreadsheet.vi"("file path (dialog if empty)"=w572, "2D data"=w577, "error in (no error)"=w576, "delimiter (\\t)"="," ("delimiter (\\t)")) -> ("error out"=w575:errorcluster)  [unwired: 10 in, 1 out]
        "Backup File I/O Error" <- w575
        n233 = Unbundle By Name(w575) -> ("code"=w570:i32)
        n234 = case shown="5" w570 {
          tunnel: w575 -> [w581 w594]
          tunnel: [w581 w593] -> w574
          tunnel: w572 -> [w582 w592]
          tunnel: w573 -> [_ w588]
          tunnel: w569 -> [w580 w589]
          tunnel: [w580 w590] -> w568
          tunnel: [w582 w583] -> w571
          frame 0, Default {
          }
          frame 5 {
            n235 = Number To Decimal String(number=w589) -> (decimal integer string=w586:string)  [unwired: 1 in]
            n236 = Strip Path(path=w592) -> (stripped path=w591:path)  [unwired: 1 out]
            n237 = Concatenate Strings(w588, "_" ("string"), w586, ".csv" ("string")) -> (w584:string)
            n238 = call <vilib>:"Clear Errors.vi"("error in (no error)"=w594) -> ("error out"=w593:errorcluster)  [unwired: 5 in, 1 out]
            n239 = Build Path(base path=w591, name or relative path=w584) -> (appended path=w583:path)
            n240 = Increment(x=w589) -> (x+1=w590:u32)
          }
        }
      }
    }
    n241 = property on="stop" class="Bool (strict)"() -> ("Value"=w515:bool)  [unwired: 2 in, 2 out]
    n242 = Unbundle By Name(w517) -> ("status"=w511:bool)
    "Backup File Error?" <- w511
    n243 = Or(x=w511, y=w515) -> (x .or. y?=w516:bool)
    "Backup File Saving?" <- "Enable?"
  }
  n244 = Merge Errors(w2, w18, w23, w20, w19, w22) -> (w17:errorcluster)
  "Overall error out" <- w17
  n245 = Unbundle By Name(w17) -> ("status"=→"Overall Error Status":bool)
  n246 = flat-sequence {
    tunnel: w17 -> [_]
    frame #0 {
      n247 = property on="stop" class="Bool (strict)"("Value"=FALSE ("stop")) -> ()  [unwired: 2 in, 2 out]
    }
  }
